vi "Has Disconnected.vi"(8 "error in (no error)":errorcluster, 11 "Buffered Subprocess in":refnum<class "Buffered Subprocess.lvclass">) -> (0 "error out":errorcluster, 2 "disconnected?":bool, 3 "Buffered Subprocess out":refnum<class "Buffered Subprocess.lvclass">)   [LabVIEW 2020, in "NI_Subprocess.lvlib" / "Buffered Subprocess.lvclass"]
uses:
  <vilib>/Subprocess/Buffered Subprocess/Buffered Subprocess.lvclass
  <vilib>/Subprocess/Buffered Subprocess/Buffered Subprocess.lvclass/Buffered Subprocess.ctl
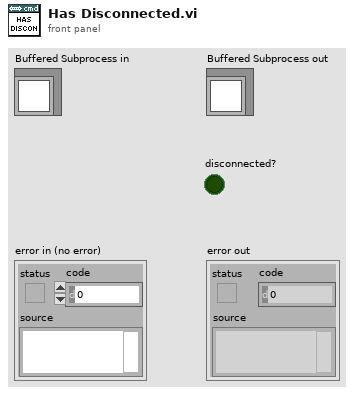
[diagram p1: front panel]
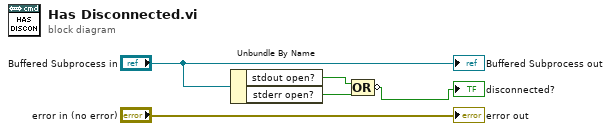
[diagram p0: block diagram]
diagram:
  n1 = Unbundle By Name("Buffered Subprocess in") -> ("stdout open?"=w2:bool, "stderr open?"=w1:bool)
  n2 = Compound Arithmetic op=OR(w2, w1) -> (invert →"disconnected?":bool)
  "error out" <- "error in (no error)"
  "Buffered Subprocess out" <- "Buffered Subprocess in"
